vi "PicowattAVS47_Open_Queue.vi"(8 "Error In":errorcluster caption="Fehler (Eingang)") -> (0 "Error Out":errorcluster caption="Fehler (Ausgang)", 2 "queue out":refnum<queue>)   [LabVIEW 2019]
uses:
  PicowattAVS47/AVS-Control-Cluster.ctl
  Global/Global Variables/Queues_global.vi
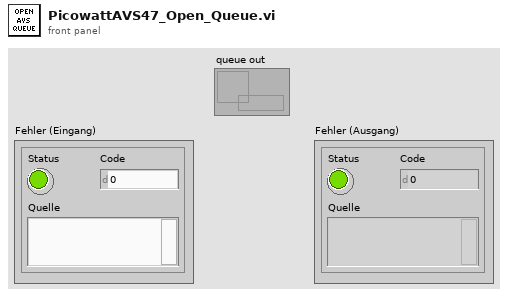
[diagram p1: front panel]
types:
  T1 = typedef "AVS-Control-Cluster.ctl" = cluster{"AVS Excitation":i16, "Auto Excitation":bool}
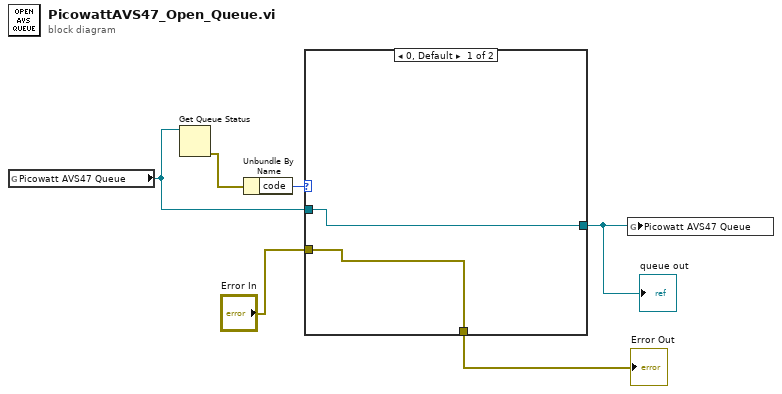
[diagram p0: block diagram]
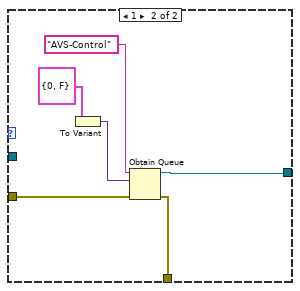
[diagram p2: hidden frame]
diagram:
  n1 = global read "Queues_global.vi" "Picowatt AVS47 Queue"() -> (w6:refnum<queue>)
  n2 = Get Queue Status(queue=w6) -> (error out=w4:errorcluster)  [unwired: 2 in, 7 out]
  n3 = Unbundle By Name(w4) -> ("code"=w5:i32)
  n4 = case shown="0, Default" w5 {
    tunnel: w6 -> [w8 _]
    tunnel: [w8 w11] -> w3
    tunnel: "Error In" -> [w7 w10]
    tunnel: [w7 w9] -> w1
    frame 0, Default {
    }
    frame 1 {
      n5 = To Variant(anything=T1 {"AVS Excitation"=0, "Auto Excitation"=FALSE} ("AVS47 Control Cluster")) -> (Variant=w13:variant)
      n6 = Obtain Queue(name (unnamed)="AVS-Control", element data type=w13, error in (no error)=w10) -> (queue out=w11:refnum<queue>, error out=w9:errorcluster)  [unwired: 2 in, 1 out]
    }
  }
  "queue out" <- w3
  "Error Out" <- w1
  n7 = global write "Queues_global.vi" "Picowatt AVS47 Queue"(w3) -> ()
